vi "Main.vi"() -> ()   [LabVIEW 2015]
uses:
  <vilib>/Utility/miscctls.llb/LVPointTypeDef.ctl
  <vilib>/Utility/miscctls.llb/LVRowAndColumnUnsignedTypeDef.ctl
  <vilib>/addons/database/Connection.llb/DB Tools Open Connec (Path).vi
  <vilib>/addons/database/Connection.llb/Conn Execute.vi
  <vilib>/addons/database/Recordset.llb/Rec Fetch Recordset Data (R).vi
  <vilib>/addons/database/Recordset.llb/Rec Destroy - Connection.vi
  <vilib>/addons/database/_DB Variant To Data/Database Variant To Data.xnode
  <vilib>/addons/database/NI_Database_API.lvlib
panel:
  out "error out":errorcluster
  in  "Value":string
  in  "Column":string(combo)
  in  "RUN 2":bool
  in  "String 2":string="update warehouse_historydata_2016.\nset lot_maker = ''\nwhere"
  in  "RUN":bool
  in  "String":string="select * from warehouse_historydata_2016.\nwhere   lot_maker like ''  and \nquantity  ='422'"
  in  "Table Control":string[][](table)
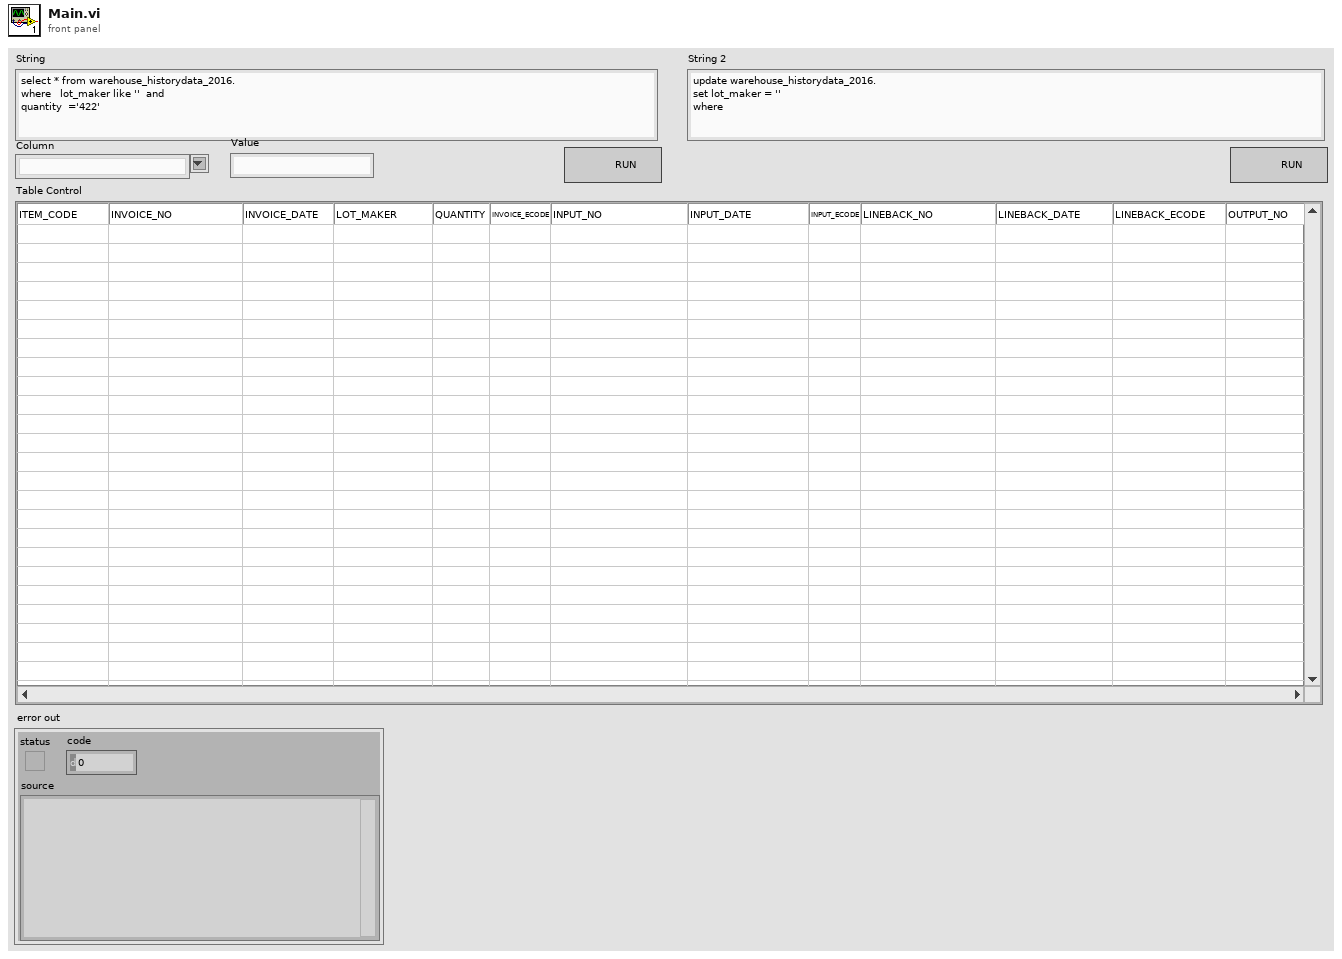
[diagram p1: front panel]
types:
  T1 = typedef "LVRowAndColumnUnsignedTypeDef.ctl" = cluster{"Row":u32, "Column":u32}
  T2 = typedef "LVPointTypeDef.ctl" = cluster{"Horizontal":i16, "Vertical":i16}
  T3 = typedef "NI_Database_API.lvlib/Conn ObjectReference.ctl" = refnum<k1>
  T4 = typedef "NI_Database_API.lvlib/Rec ObjectReference.ctl" = refnum<k1>
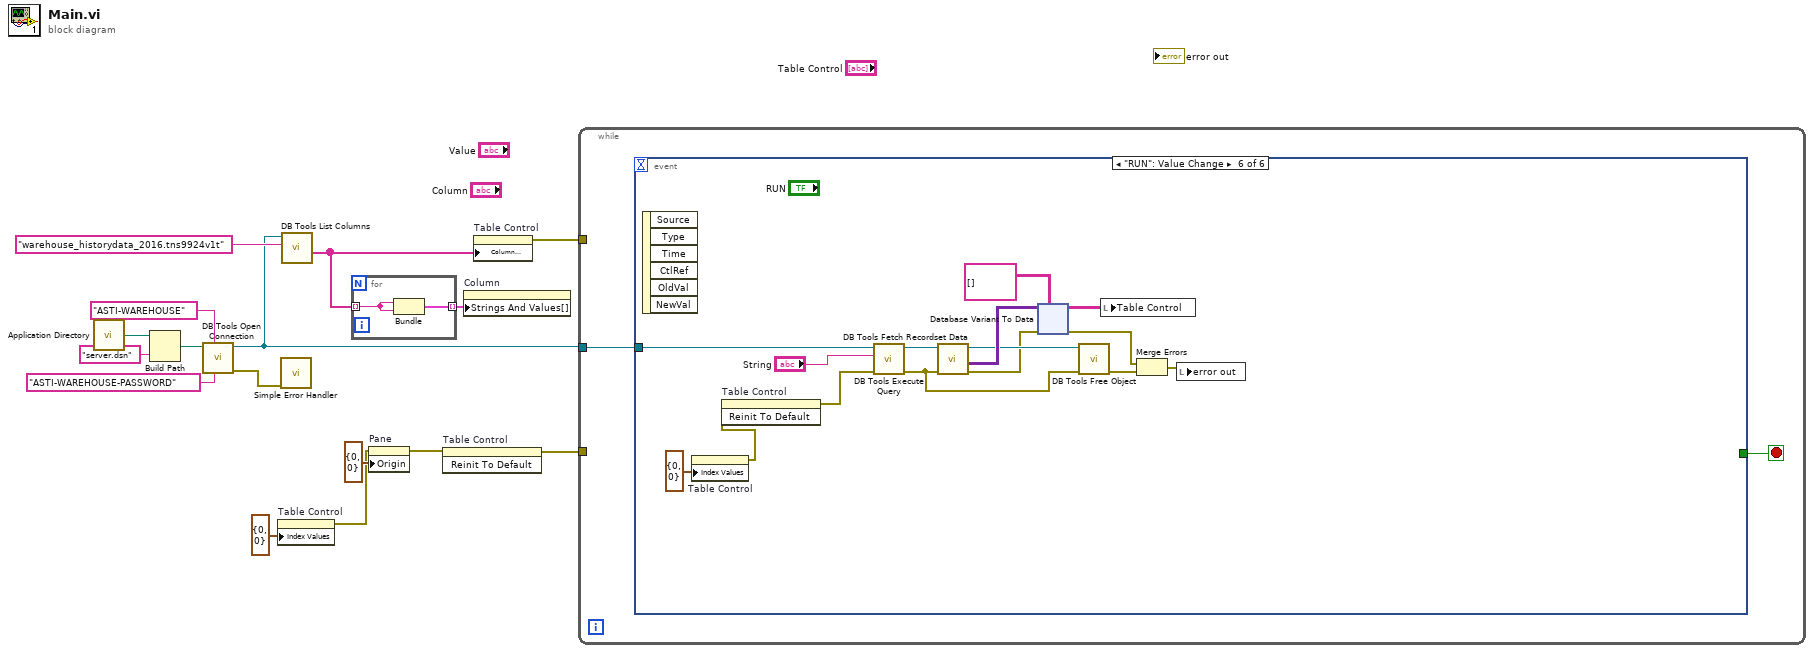
[diagram p0: block diagram]
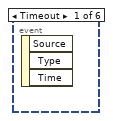
[diagram p2: hidden frame]
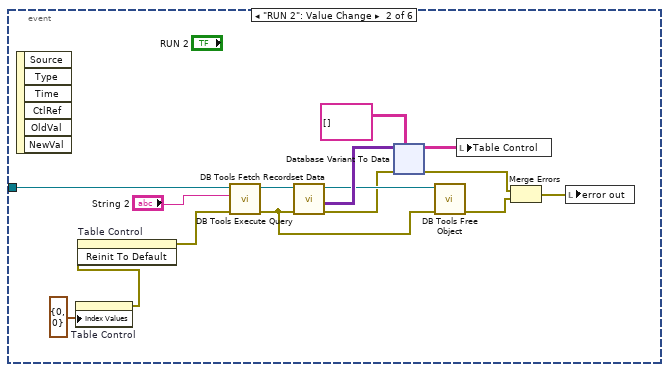
[diagram p3: hidden frame]
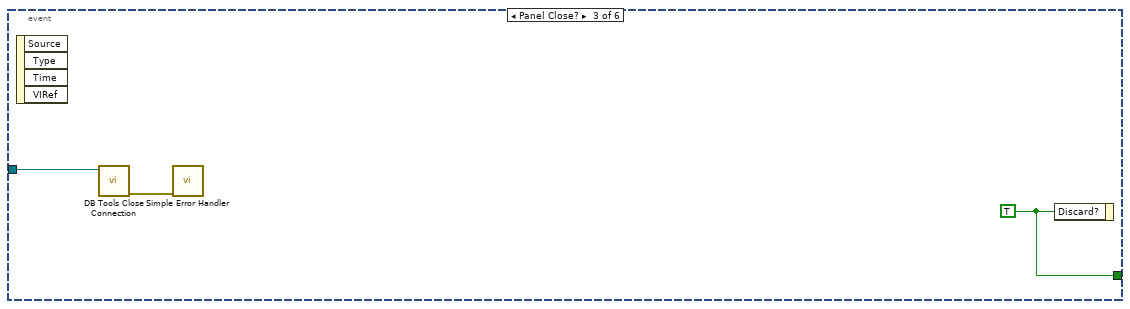
[diagram p4: hidden frame]
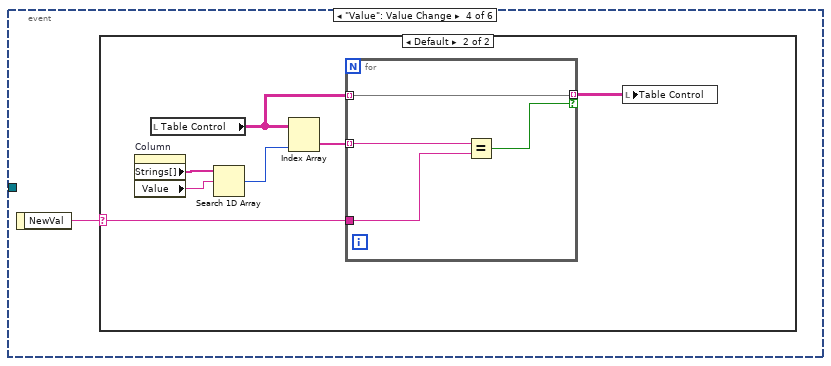
[diagram p5: hidden frame]
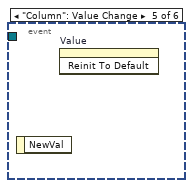
[diagram p7: hidden frame]
diagram:
  n1 = call <vilib>:"Application Directory.vi"() -> ("Application Directory"=w13:path)
  n2 = Build Path(base path=w13, name or relative path="server.dsn") -> (appended path=w14:path)
  n3 = call-poly <vilib>:"DB Tools Open Connection.vi"("password"="ASTI-WAREHOUSE-PASSWORD", "userID"="ASTI-WAREHOUSE", "connection information"=w14) -> ("error out"=w11:errorcluster, "connection reference"=w8:T3)  [unwired: 5 in]
  n4 = property on="Table Control" class="Tbl (strict)"("Index Values"=T1 {"Row"=0, "Column"=0}) -> (error out=w2:errorcluster)  [unwired: 2 in, 1 out]
  n5 = call <vilib>:"Simple Error Handler.vi"("error in (no error)"=w11) -> ()  [unwired: 4 in, 5 out]
  n6 = call <vilib>:"DB Tools List Columns.vi"("table"="warehouse_historydata_2016.tns9924v1t", "connection reference"=w8) -> ("columns"=w7:string[])  [unwired: 2 in, 3 out]
  n7 = for {
    tunnel: w7 -> [w18] mode=indexing
    tunnel: [w17] -> w6 mode=indexing
    n8 = Bundle("String"=w18, "String"=w18) -> (w17:cluster{"String":string, "String":string})  [unwired: 1 in]
  }
  n9 = property on="Pane" class="Pane"(error in=w2, "Origin"=T2 {"Horizontal"=0, "Vertical"=0}) -> (error out=w3:errorcluster)  [unwired: 1 in, 1 out]
  n10 = invoke on="Table Control" class="Tbl (strict)" method="Reinit To Default"(error in=w3) -> (error out=w5:errorcluster)  [unwired: 2 in, 2 out]
  n11 = property on="Column" class="CmbBox"("Strings And Values[]"=w6) -> ()  [unwired: 2 in, 2 out]
  n12 = property on="Table Control" class="Tbl (strict)"("Column Headers[]"=w7) -> (error out=w10:errorcluster)  [unwired: 2 in, 1 out]
  n13 = while {
    tunnel: w8 -> [w20]
    tunnel: w10 -> [_]
    tunnel: w5 -> [_]
    stop <- w19 stop-if-true
    n14 = event shown="[5] \"RUN\": Value Change" {
      selector: _ -> [_ _ _ _ _ _]
      dyn-events: _ -> [_ _ _ _ _ _]
      timeout: _ -> [_ _ _ _ _ _]
      tunnel: w20 -> [_ w29 w81 _ _ w108]
      tunnel: [_ _ w82 _ _ _] -> w19
      event Timeout {
        n15 = event-data() -> ()  [unwired: 1 in, 3 out]
      }
      event "RUN 2": Value Change {
        n16 = event-data() -> ()  [unwired: 1 in, 6 out]
        n17 = property on="Table Control" class="Tbl (strict)"("Index Values"=T1 {"Row"=0, "Column"=0}) -> (error out=w21:errorcluster)  [unwired: 2 in, 1 out]
        n18 = invoke on="Table Control" class="Tbl (strict)" method="Reinit To Default"(error in=w21) -> (error out=w30:errorcluster)  [unwired: 2 in, 2 out]
        n19 = call-poly <vilib>:"DB Tools Execute Query.vi"("error in (no error)"=w30, "SQL query"="String 2", "connection reference"=w29) -> ("error out"=w27:errorcluster, "recordset reference"=w35:T4)  [unwired: 5 in]
        n20 = call-poly <vilib>:"DB Tools Fetch Recordset Data.vi"("error in (no error)"=w27, "recordset reference"=w35) -> ("error out"=w26:errorcluster, "recordset data"=w33:variant[][], "recordset reference out"=w32:T4)  [unwired: 3 in]
        n21 = xnode "Database Variant To Data"("database variant"=w33, "error in (no error)"=w26, "type"=string[][] []) -> ("data"=w31:string[][], "error out"=w23:errorcluster)
        n22 = call-poly <vilib>:"DB Tools Free Object.vi"("error in (no error)"=w27, "recordset reference"=w32) -> ("error out"=w24:errorcluster)  [unwired: 8 in, 1 out]
        n23 = local write "Table Control"(w31) -> ()
        n24 = Merge Errors(w23, w24) -> (w25:errorcluster)
        n25 = local write "error out"(w25) -> ()
      }
      event Panel Close? {
        w82 = TRUE ("Discard?")
        n26 = event-data() -> ()  [unwired: 1 in, 4 out]
        n27 = call <vilib>:"DB Tools Close Connection.vi"("connection reference"=w81) -> ("error out"=w80:errorcluster)  [unwired: 6 in]
        n28 = call <vilib>:"Simple Error Handler.vi"("error in (no error)"=w80) -> ()  [unwired: 4 in, 5 out]
        n29 = event-data("Discard?"=w82) -> ()  [unwired: 1 in, 1 out]
      }
      event "Value": Value Change {
        n30 = event-data() -> ("NewVal"=w83:string)  [unwired: 1 in]
        n31 = case shown="Default" w83 {
          selector: w83 -> [_ w86]
          frame "" {
          }
          frame Default {
            n32 = property on="Column" class="CmbBox"() -> ("Strings[]"=w90:string[], "Value"=w89:string)  [unwired: 2 in, 2 out]
            n33 = local read "Table Control"() -> (w85:string[][])
            n34 = Search 1D Array(1D array=w90, element=w89) -> (index of element=w88:i32)  [unwired: 1 in]
            n35 = Index Array(array=w85, index (col)=w88) -> (element=w87:string[])  [unwired: 1 in]
            n36 = for {
              tunnel: w87 -> [w94] mode=indexing
              tunnel: w86 -> [w93]
              tunnel: w85 -> [w92] mode=indexing
              tunnel: [w92] -> w84 mode=indexing if=w91
              n37 = Equal?(x=w94, y=w93) -> (x = y?=w91:bool)
            }
            n38 = local write "Table Control"(w84) -> ()
          }
        }
      }
      event "Column": Value Change {
        n39 = event-data() -> ()  [unwired: 1 in, 1 out]
        n40 = invoke on="Value" class="Str" method="Reinit To Default"() -> ()  [unwired: 3 in, 3 out]
      }
      event "RUN": Value Change {
        n41 = event-data() -> ()  [unwired: 1 in, 6 out]
        n42 = property on="Table Control" class="Tbl (strict)"("Index Values"=T1 {"Row"=0, "Column"=0}) -> (error out=w95:errorcluster)  [unwired: 2 in, 1 out]
        n43 = invoke on="Table Control" class="Tbl (strict)" method="Reinit To Default"(error in=w95) -> (error out=w102:errorcluster)  [unwired: 2 in, 2 out]
        n44 = call-poly <vilib>:"DB Tools Execute Query.vi"("error in (no error)"=w102, "SQL query"="String", "connection reference"=w108) -> ("error out"=w100:errorcluster, "recordset reference"=w107:T4)  [unwired: 5 in]
        n45 = call-poly <vilib>:"DB Tools Fetch Recordset Data.vi"("error in (no error)"=w100, "recordset reference"=w107) -> ("error out"=w101:errorcluster, "recordset data"=w105:variant[][], "recordset reference out"=w104:T4)  [unwired: 3 in]
        n46 = xnode "Database Variant To Data"("database variant"=w105, "error in (no error)"=w101, "type"=string[][] []) -> ("data"=w103:string[][], "error out"=w97:errorcluster)
        n47 = call-poly <vilib>:"DB Tools Free Object.vi"("error in (no error)"=w100, "recordset reference"=w104) -> ("error out"=w99:errorcluster)  [unwired: 8 in, 1 out]
        n48 = local write "Table Control"(w103) -> ()
        n49 = Merge Errors(w97, w99) -> (w98:errorcluster)
        n50 = local write "error out"(w98) -> ()
      }
    }
  }
